vi "Receive Value Change Event.vi"(8 "error in (no error)":errorcluster, 10 "ValueChangeMsg":refnum<class "ValueChangeMsg.lvclass">, 11 "OneButtonDialogBox in":refnum<class "KeypadDialogBox.lvclass">) -> (0 "error out":errorcluster, 3 "OneButtonDialogBox out":refnum<class "KeypadDialogBox.lvclass">)   [LabVIEW 2017, in "KeypadDialogBox.lvlib" / "KeypadDialogBox.lvclass"]
uses:
  KeypadDialogBox.lvclass
  C:/Program Files (x86)/National Instruments/LabVIEW 2017/vi.lib/ActorFramework/Actor/Actor.lvclass
  Framework/ActorEvents/IEventAggregator Messages/ValueChangeMsg/ValueChangeMsg.lvclass
  Framework/ActorEvents/IEventAggregator Messages/ValueChangeMsg/ValueChangeMsg.lvclass/ValueChangeMsg.ctl
  <vilib>/ActorFramework/Actor/Actor.lvclass/Actor.ctl
  <vilib>/ActorFramework/Message Enqueuer/Message Enqueuer.lvclass/Message Enqueuer.ctl
  KeypadDialogBox.lvclass/KeypadDialogBox.ctl
  <vilib>/ActorFramework/Message Enqueuer/Init from Existing Queue.vi
  <vilib>/ActorFramework/Message Enqueuer/Enqueue.vi
  <vilib>/ActorFramework/Stop Msg/Stop Msg.lvclass
  C:/Program Files (x86)/National Instruments/LabVIEW 2017/vi.lib/ActorFramework/Message/Message.lvclass
  <vilib>/ActorFramework/Message Priority Queue/Priority Enqueue.vi
  <vilib>/ActorFramework/Message Enqueuer/Message Enqueuer.lvclass
  Framework/IMediator/ITransport/ITransport.lvclass
  <vilib>/ActorFramework/Actor/Actor.lvclass
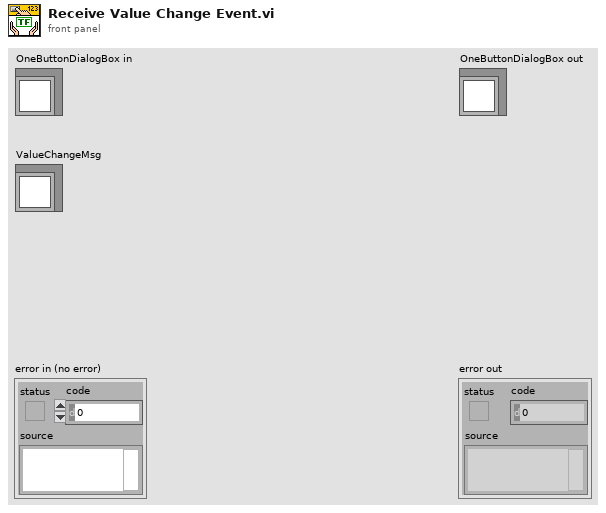
[diagram p1: front panel]
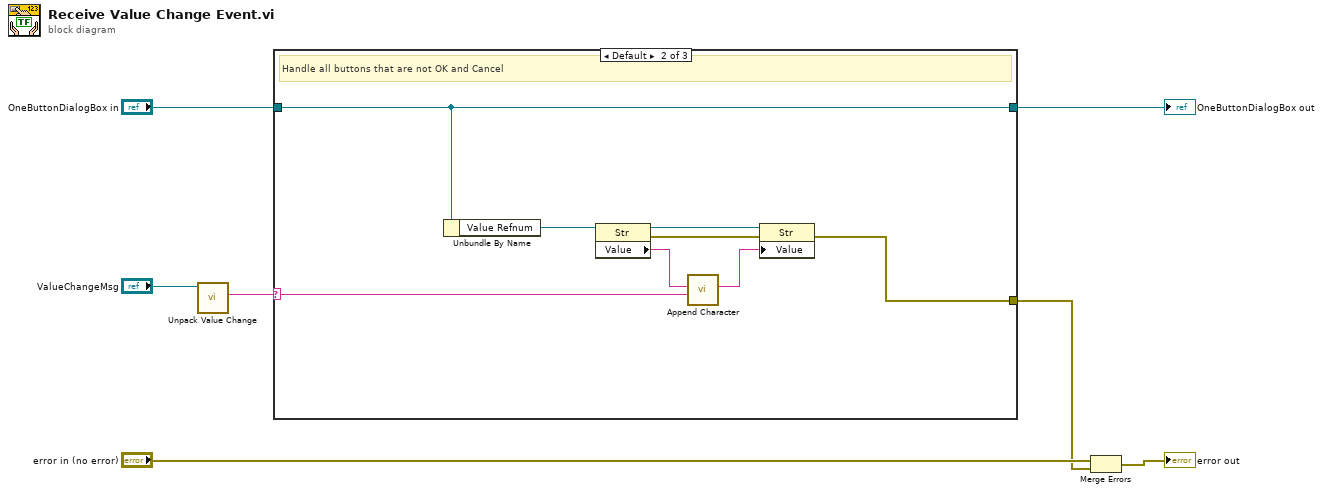
[diagram p0: block diagram]
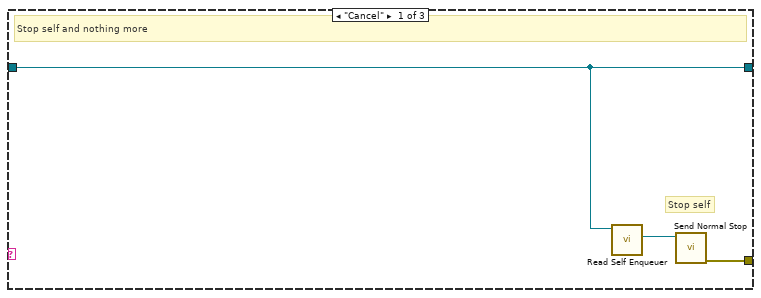
[diagram p2: hidden frame]
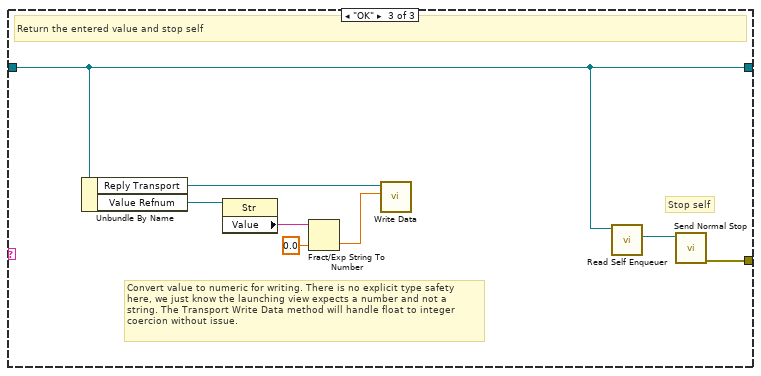
[diagram p3: hidden frame]
diagram:
  n1 = call "Unpack Value Change.vi"("ValueChangeMsg"="ValueChangeMsg") -> ("Control Label"=w1:string)  [unwired: 6 in, 4 out]
  n2 = case shown="Default" w1 {
    selector: w1 -> [_ w15 _]
    tunnel: "OneButtonDialogBox in" -> [w8 w18 w25]
    tunnel: [w8 w18 w25] -> w3
    tunnel: [w9 w12 w24] -> w2
    frame "Cancel" {
      # "Stop self"
      # "Stop self and nothing more"
      n3 = call <vilib>:"Read Self Enqueuer.vi"("Actor"=w8) -> ("Self Enqueuer"=w10:refnum<class "Message Enqueuer.lvclass">)  [unwired: 10 in]
      n4 = call <vilib>:"Send Normal Stop.vi"("Message Enqueuer"=w10) -> ("error out"=w9:errorcluster)  [unwired: 10 in]
    }
    frame Default {
      # "Handle all buttons that are not OK and Cancel"
      n5 = Unbundle By Name(w18) -> ("Value Refnum"=w17:refnum<vi>)
      n6 = property class="Str"(reference=w17) -> (reference out=w14:refnum<vi>, error out=w11:errorcluster, "Value"=w16:string)  [unwired: 1 in]
      n7 = call "Append Character.vi"("Character"=w15, "String In"=w16) -> ("String Out"=w13:string)  [unwired: 9 in]
      n8 = property class="Str"(reference=w14, error in=w11, "Value"=w13) -> (error out=w12:errorcluster)  [unwired: 1 out]
    }
    frame "OK" {
      # "Convert value to numeric for writing. There is no explicit type safety\nhere, we just know the launching view expects a number and not a\nstring. The Transport Write Data method will handle float to integer\ncoercion without issue."
      # "Stop self"
      # "Return the entered value and stop self"
      n9 = Unbundle By Name(w25) -> ("Reply Transport"=w20:refnum<class "ITransport.lvclass">, "Value Refnum"=w23:refnum<vi>)
      n10 = property class="Str"(reference=w23) -> ("Value"=w22:string)  [unwired: 1 in, 2 out]
      n11 = Fract/Exp String To Number(string=w22, default (0 dbl)=0.0 ("default (0 DBL)")) -> (number=w19:dbl)  [unwired: 2 in, 1 out]
      n12 = call-dynamic "Write Data.vi"("Value"=w19, "ITransport in"=w20) -> ()  [unwired: 8 in, 2 out]
      n13 = call <vilib>:"Read Self Enqueuer.vi"("Actor"=w25) -> ("Self Enqueuer"=w26:refnum<class "Message Enqueuer.lvclass">)  [unwired: 10 in]
      n14 = call <vilib>:"Send Normal Stop.vi"("Message Enqueuer"=w26) -> ("error out"=w24:errorcluster)  [unwired: 10 in]
    }
  }
  "OneButtonDialogBox out" <- w3
  n15 = Merge Errors("error in (no error)", w2) -> (→"error out":errorcluster)
